vi "DATAExport.vi"(0 "additonal Mass[g]":dbl, 1 "Subject ID":dbl, 2 "Humidity":dbl, 3 "Data Export":bool, 5 "SpeedLaser":dbl, 7 "Impactor ID":dbl, 9 "Exp_in":dbl, 11 "error in (no error)":errorcluster, 12 "Username":string, 13 "Impact Speed":dbl) -> (4 "Exp_id":i32, 15 "error out":errorcluster)   [LabVIEW 2020]
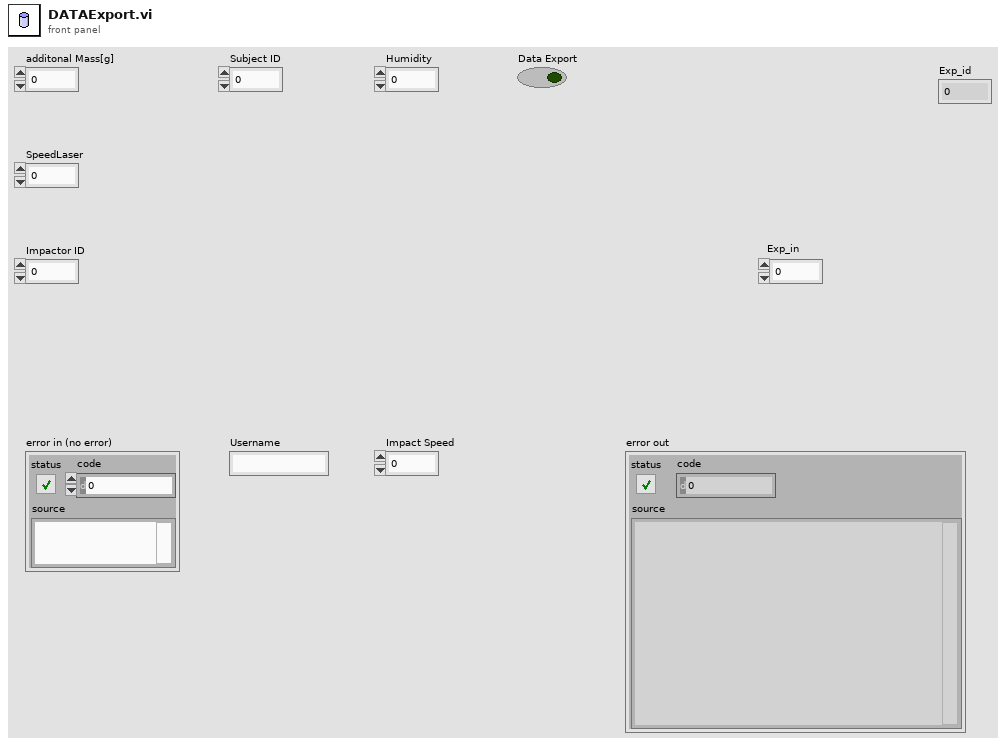
[diagram p1: front panel]
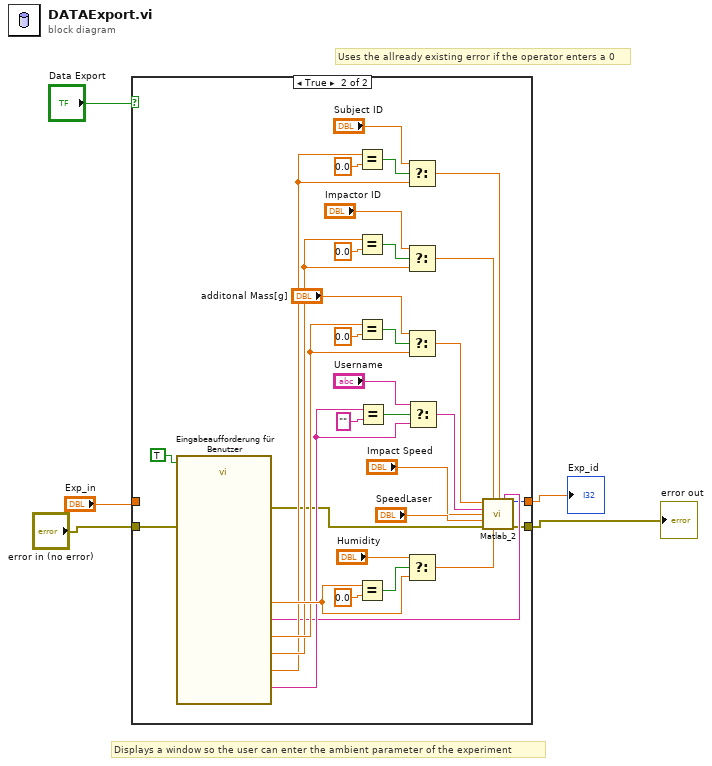
[diagram p0: block diagram]
diagram:
  # "Uses the allready existing error if the operator enters a 0"
  # "Displays a window so the user can enter the ambient parameter of the experiment"
  n1 = case shown="True" "Data Export" {
    tunnel: "error in (no error)" -> [w7 w27]
    tunnel: [w7 w9] -> w3
    tunnel: [w6 w8] -> w2
    tunnel: "Exp_in" -> [w6 _]
    frame False {
    }
    frame True {
      n2 = call "Eingabeaufforderung für Benutzer"("Enable"=TRUE, "error in (no error)"=w27) -> ("username"=w24:string, "Impactor_id"=w31:dbl, "Subject_id"=w29:dbl, "additional Mass [g]"=w33:dbl, "Comment"=w17:string, "Humidity [%]"=w38:dbl, "error out"=w18:errorcluster)  [unwired: 10 in, 1 out]
      n3 = Equal?(x=w29, y=0.0) -> (x = y?=w30:bool)
      n4 = Equal?(x=w31, y=0.0) -> (x = y?=w32:bool)
      n5 = Equal?(x=w33, y=0.0) -> (x = y?=w34:bool)
      n6 = Equal?(x=w38, y=0.0) -> (x = y?=w39:bool)
      n7 = Equal?(x=w24, y="") -> (x = y?=w26:bool)
      n8 = Select(t="Subject ID", s=w30, f=w29) -> (s? t:f=w10:dbl)
      n9 = Select(t="Impactor ID", s=w32, f=w31) -> (s? t:f=w11:dbl)
      n10 = Select(t="additonal Mass[g]", s=w34, f=w33) -> (s? t:f=w12:dbl)
      n11 = Select(t="Humidity", s=w39, f=w38) -> (s? t:f=w16:dbl)
      n12 = Select(t="Username", s=w26, f=w24) -> (s? t:f=w13:string)
      n13 = call "Matlab_2.vi"("additonal Mass[g]"=w12, "Subject ID"=w11, "Impactor ID"=w10, "comment"=w17, "loginName"=w13, "Impact Speed"="Impact Speed", "Pendel Velocity"="SpeedLaser", "Fehler (Eingang, kein Fehler)"=w18, "Humidity"=w16) -> ("Exp_id"=w8:i32, "Fehler (Ausgang)"=w9:errorcluster)  [unwired: 5 in]
    }
  }
  "error out" <- w3
  "Exp_id" <- w2
